vi "Begin.vi"() -> (0 "error out":errorcluster)   [LabVIEW 2013]
doc: "Called before other user functions, this VI is expected to open initial I/O refnums, load in file data, and do all program initialization. Notice that the <B>error out</B> terminal is simply used for data flow. Wiring it to other structures or subVIs ensures that this VI runs first."
uses:
  <vilib>/Rock Robotics/WPI/Joystick/WPI_JoystickDeviceEnum.ctl
  <vilib>/Rock Robotics/SystemInterfaces/Typedef/FPGA_TypedefDigitalModule.ctl
  <vilib>/Rock Robotics/SystemInterfaces/DIO/FPGA_DIOChannel.ctl
  <vilib>/Rock Robotics/SystemInterfaces/DIO/FPGA_DIORelayChannel.ctl
  <vilib>/Rock Robotics/SystemInterfaces/Typedef/FPGA_TypedefSolenoidModule.ctl
  <vilib>/Rock Robotics/WPI/Solenoid/WPI_SolenoidChannel.ctl
  <vilib>/Rock Robotics/WPI/Solenoid/WPI_SolenoidValue.ctl
  <vilib>/Rock Robotics/SystemInterfaces/DIO/FPGA_DIOPWMChannel.ctl
  <vilib>/Rock Robotics/WPI/Encoder/WPI_EncoderType.ctl
  <vilib>/Rock Robotics/WPI/Solenoid/WPI_SolenoidOpenDouble.vi
  <vilib>/Rock Robotics/WPI/Solenoid/WPI_SolenoidSetEnum.vi
  <vilib>/Rock Robotics/WPI/Counter/WPI_CounterDigitalInputToDigitalSource.vi
  <vilib>/Rock Robotics/WPI/RobotDrive/WPI_RobotDriveOpen2MotorWithVictor.vi
  <vilib>/Rock Robotics/WPI/MotorControl/WPI_MotorControlOpen Jaguar.vi
  <vilib>/Rock Robotics/WPI/MotorControl/WPI_MotorControlOpen Victor.vi
  <vilib>/Rock Robotics/WPI/Compressor/WPI_CompressorGetSetRefNum.vi
  <vilib>/Rock Robotics/WPI/Camera/WPI_CameraImageSize.ctl
  <vilib>/Rock Robotics/WPI/Camera/WPI_CameraWhite Balance Values.ctl
  <vilib>/Rock Robotics/WPI/Camera/WPI_CameraExposure Values.ctl
  <vilib>/Rock Robotics/WPI/Camera/WPI_CameraFrameRate.ctl
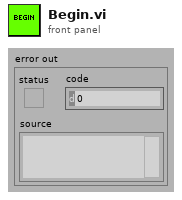
[diagram p1: front panel]
types:
  T1 = typedef "FPGA_DIOChannel.ctl" = enum8{"DIO 1", "DIO 2", "DIO 3", "DIO 4", "DIO 5", "DIO 6", "DIO 7", "DIO 8", "DIO 9", "DIO 10", "DIO 11", "DIO 12", "DIO 13", "DIO 14", "Invalid"}
  T2 = typedef "WPI_SolenoidChannel.ctl" = enum8{"Solenoid 1", "Solenoid 2", "Solenoid 3", "Solenoid 4", "Solenoid 5", "Solenoid 6", "Solenoid 7", "Solenoid 8", "Invalid"}
  T3 = typedef "FPGA_DIOPWMChannel.ctl" = enum8{"PWM 1", "PWM 2", "PWM 3", "PWM 4", "PWM 5", "PWM 6", "PWM 7", "PWM 8", "PWM 9", "PWM 10", "Invalid"}
  T4 = typedef "WPI_EncoderType.ctl" = enum16{"1x", "2x", "4x"}
  T5 = typedef "WPI_SolenoidValue.ctl" = enum16{"Off", "On", "Forward", "Reverse"}
  T6 = typedef "FPGA_TypedefSolenoidModule.ctl" = enum16{"Solenoid Module 1", "Solenoid Module 2"}
  T7 = typedef "FPGA_DIORelayChannel.ctl" = enum8{"Relay 1", "Relay 2", "Relay 3", "Relay 4", "Relay 5", "Relay 6", "Relay 7", "Relay 8", "Invalid"}
  T8 = typedef "WPI_JoystickDeviceEnum.ctl" = enum16{"USB 1", "USB 2", "USB 3", "USB 4", "Kinect 1", "Kinect 2"}
  T9 = typedef "FPGA_TypedefDigitalModule.ctl" = enum16{"Digital Module 1", "Digital Module 2"}
  T10 = typedef "WPI_CameraFrameRate.ctl" = u32
  T11 = typedef "WPI_CameraExposure Values.ctl" = enum16{"Auto", "Flicker-free 50 Hz", "Flicker-free 60 Hz", "Hold current"}
  T12 = typedef "WPI_CameraWhite Balance Values.ctl" = enum16{"Auto", "Fixed indoor", "Fixed outdoor 1", "Fixed outdoor 2", "Fixed fluorescent 1", "Fixed fluorescent 2", "Hold current"}
  T13 = typedef "WPI_CameraImageSize.ctl" = enum16{"640x480", "320x240", "160x120"}
  T14 = typedef "WPI_CameraDevRef.ctl" = cluster{"Camera Address":string, "CameraStatus":errorcluster, "Acquire Image Notifier":refnum<notifier>}
  T15 = typedef "WPI_DigitalInputDevRef.ctl" = cluster{"DevStatus":errorcluster, "DIO Channel":T1, "Digital Module":T9}
  T16 = typedef "WPI_MotorControlDeviceRef.ctl" = cluster{"DeviceStatus":errorcluster, "Type":enum16{"PWM", "CAN"}, "PWM":cluster{"Digital Module":T9, "PWM Channel":T3, "DeadBand":T17}, "CAN":cluster{"Device Number":u8, "Control Mode":T18, "Semaphore":T19, "Max Vout":dbl}, "Invert":bool, "TransformRef":T20, "InvTransformRef":T20}
  T17 = typedef "WPI_PWMDeadband.ctl" = cluster{"Name":string, "maxPositivePwm":i32, "minPositivePwm":i32, "centerPwm":i32, "maxNegativePwm":i32, "minNegativePwm":i32, "angularRange":u16}
  T18 = typedef "WPI_CANJaguar_ControlMode.ctl" = enum8{"Percent VBus", "Current", "Speed", "Position", "Voltage"}
  T19 = typedef "Semaphore RefNum" = refnum<k1>
  T20 = typedef "WPI_PWMTransform_ConPane.ctl" = refnum<vi>
  T21 = typedef "WPI_SolenoidDevRef.ctl" = cluster{"DevStatus":errorcluster, "Solenoid Module":T6, "Forward Solenoid Channel":T2, "Reverse Solenoid Channel":T2}
  T22 = typedef "FPGA_CounterEncoderSourceConvertionLVSourceType.ctl" = cluster{"DevStatus":errorcluster, "AnalogTriggerMode?":bool, "DigitalMode":cluster{"Digital Module":T9, "DIO Channel":T23}, "AnalogTriggerMode":cluster{"AnalogTriggerIndex":T24, "OutputType":T25}}
  T23 = typedef "FPGA_DIODigitalSourceChannel.ctl" = enum8{"DIO 1", "DIO 2", "DIO 3", "DIO 4", "DIO 5", "DIO 6", "DIO 7", "DIO 8", "DIO 9", "DIO 10", "DIO 11", "DIO 12", "DIO 13", "DIO 14", "Disabled"}
  T24 = typedef "FPGA_AnalogTriggerIndex.ctl" = enum8{"Trig 0", "Trig 1", "Trig 2", "Trig 3", "Trig 4", "Trig 5", "Trig 6", "Trig 7", "Invalid"}
  T25 = typedef "FPGA_AnalogTriggerOutType.ctl" = enum16{"InWindow", "TriggerState", "Rising", "Falling"}
  T26 = typedef "WPI_CompressorDevRef.ctl" = cluster{"DevStatus":errorcluster, "DigitalInputDevRef":T15, "RelayDevRef":T27}
  T27 = typedef "WPI_RelayDevRef.ctl" = cluster{"DevStatus":errorcluster, "Relay Channel":T7, "Digital Module":T9, "Relay Direction":T28}
  T28 = typedef "WPI_RelayDirection.ctl" = enum16{"Both directions", "Forward only", "Reverse only"}
  T29 = typedef "WPI_RobotDriveDevRef.ctl" = cluster{"DevStatus":errorcluster, "Motors[]":T16[], "Square Inputs":bool, "Max Output":dbl, "Isochronous":bool}
  T30 = typedef "WPI_EncoderDevRef.ctl" = cluster{"DevStatus":errorcluster, "EncoderIndex":T31, "CounterIndex":T32, "DistancePerCount":dbl, "Decoding Type":T4}
  T31 = typedef "FPGA_EncoderIdx.ctl" = enum8{"Enc 0", "Enc 1", "Enc 2", "Enc 3", "Invalid"}
  T32 = typedef "FPGA_CounterCtrSystemIndex.ctl" = enum8{"Ctr 0", "Ctr 1", "Ctr 2", "Ctr 3", "Ctr 4", "Ctr 5", "Ctr 6", "Ctr 7", "Invalid"}
  T33 = typedef "WPI_JoystickDevRef.ctl" = cluster{"Device":T8}
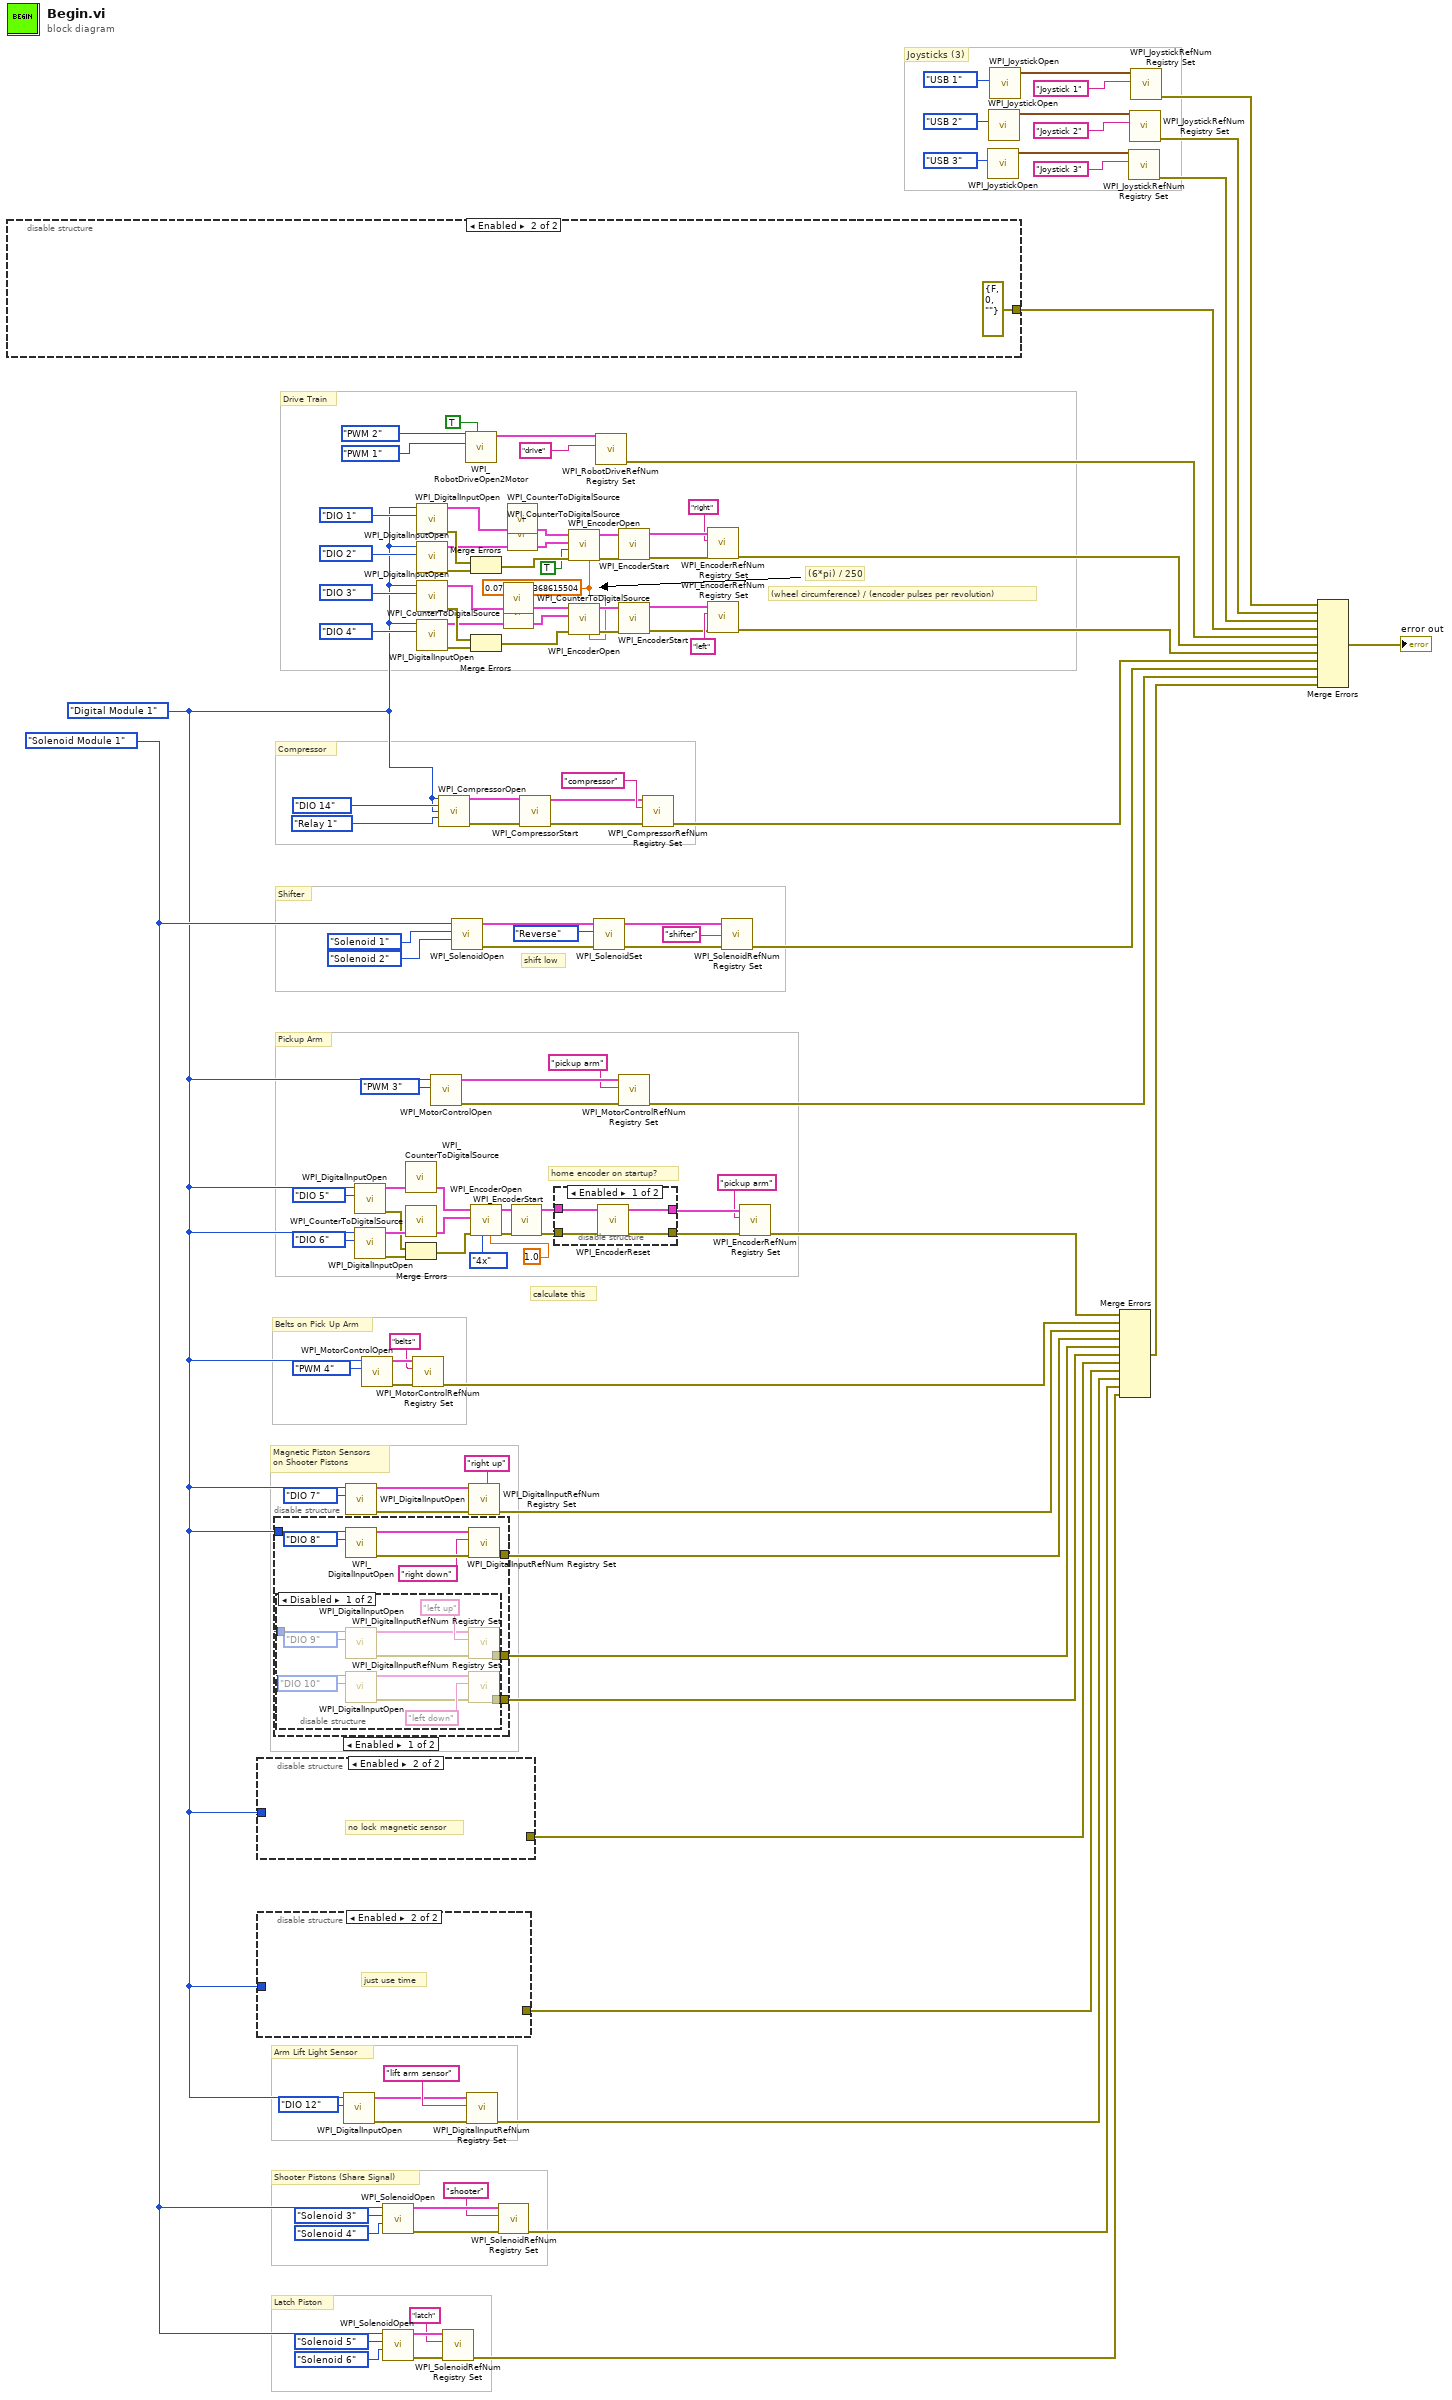
[diagram p0: block diagram]
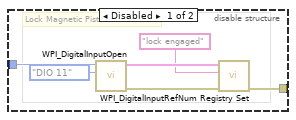
[diagram p2: hidden frame]
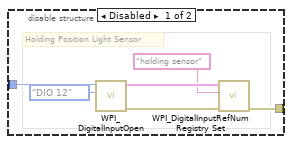
[diagram p5: hidden frame]
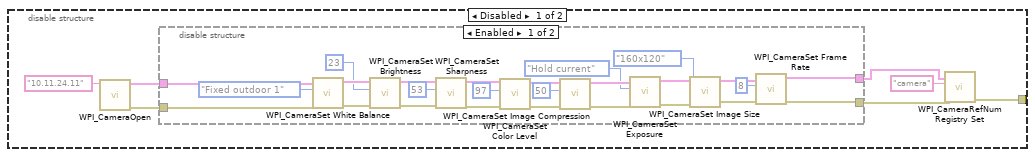
[diagram p7: hidden frame]
diagram:
  w72 = 0.07539822368615504 ("DistancePerCount")
  w13 = FPGA_TypedefSolenoidModule."Solenoid Module 1" ("Solenoid Module (Module 1)")
  w6 = FPGA_TypedefDigitalModule."Digital Module 1" ("Digital Module (Module 1)")
  # "Arm Lift Light Sensor"
  # "Joysticks (3)"
  # "Latch Piston"
  # "Shooter Pistons (Share Signal)"
  # "Magnetic Piston Sensors\non Shooter Pistons"
  # "Belts on Pick Up Arm"
  # "calculate this"
  # "Pickup Arm"
  # "home encoder on startup?"
  # "Shifter"
  # "Compressor"
  # "Drive Train"
  # "shift low"
  # "(wheel circumference) / (encoder pulses per revolution)"
  # "(6*pi) / 250"
  n1 = disable-structure shown="Enabled" {
    disable-tunnel: [w129 errorcluster {"status"=FALSE, "code"=0, "source"=""} ("error out")] -> w116
    frame Disabled {
      n2 = call <vilib>:"WPI_CameraOpen.vi"("Camera Address"="10.11.24.11") -> ("error out"=w131:errorcluster, "CameraDevRef"=w133:T14)  [unwired: 9 in]
      n3 = disable-structure shown="Enabled" {
        disable-tunnel: w133 -> [w159 w163]
        disable-tunnel: [w137 w163] -> w132
        disable-tunnel: w131 -> [w146 w162]
        disable-tunnel: [w136 w162] -> w130
        frame Enabled {
          n4 = call <vilib>:"WPI_CameraSet White Balance.vi"("error in (no error)"=w146, "White Balance"=WPI_CameraWhite_Balance_Values."Fixed outdoor 1", "CameraDevRef"=w159) -> ("error out"=w147:errorcluster, "CameraDevRef Out"=w158:T14)  [unwired: 7 in]
          n5 = call <vilib>:"WPI_CameraSet Brightness.vi"("error in (no error)"=w147, "Brightness"=23, "CameraDevRef"=w158) -> ("error out"=w148:errorcluster, "CameraDevRef Out"=w157:T14)  [unwired: 7 in]
          n6 = call <vilib>:"WPI_CameraSet Sharpness.vi"("error in (no error)"=w148, "Sharpness"=53, "CameraDevRef"=w157) -> ("error out"=w149:errorcluster, "CameraDevRef Out"=w156:T14)  [unwired: 7 in]
          n7 = call <vilib>:"WPI_CameraSet Color Level.vi"("error in (no error)"=w149, "Color Level"=97, "CameraDevRef"=w156) -> ("error out"=w150:errorcluster, "CameraDevRef Out"=w155:T14)  [unwired: 7 in]
          n8 = call <vilib>:"WPI_CameraSet Image Compression.vi"("error in (no error)"=w150, "Compression"=50, "CameraDevRef"=w155) -> ("error out"=w161:errorcluster, "CameraDevRef Out"=w160:T14)  [unwired: 7 in]
          n9 = call <vilib>:"WPI_CameraSet Exposure.vi"("error in (no error)"=w161, "Exposure"=WPI_CameraExposure_Values."Hold current", "CameraDevRef"=w160) -> ("error out"=w151:errorcluster, "CameraDevRef Out"=w154:T14)  [unwired: 7 in]
          n10 = call <vilib>:"WPI_CameraSet Image Size.vi"("error in (no error)"=w151, "Image Size"=WPI_CameraImageSize."160x120", "CameraDevRef"=w154) -> ("error out"=w152:errorcluster, "CameraDevRef Out"=w153:T14)  [unwired: 7 in]
          n11 = call <vilib>:"WPI_CameraSet Frame Rate.vi"("error in (no error)"=w152, "Frame Rate (fps)"=T10 8, "CameraDevRef"=w153) -> ("error out"=w136:errorcluster, "CameraDevRef Out"=w137:T14)  [unwired: 7 in]
        }
        frame Disabled {
        }
      }
      n12 = call <vilib>:"WPI_CameraRefNum Registry Set.vi"("error in (no error)"=w130, "refnum name"="camera", "CameraDevRef"=w132) -> ("error out"=w129:errorcluster)  [unwired: 7 in, 1 out]
    }
    frame Enabled {
    }
  }
  n13 = disable-structure shown="Enabled" {
    disable-tunnel: w6 -> [w166 _]
    disable-tunnel: [w165 _] -> w1
    frame Disabled {
      # "Lock Magnetic Piston Sensor"
      n14 = call <vilib>:"WPI_DigitalInputOpen.vi"("DIO Channel"=FPGA_DIOChannel."DIO 11", "Digital Module (Module 1)"=w166) -> ("error out"=w169:errorcluster, "DigitalInputDevRef"=w168:T15)  [unwired: 8 in]
      n15 = call <vilib>:"WPI_DigitalInputRefNum Registry Set.vi"("error in (no error)"=w169, "refnum name"="lock engaged", "DigitalInputDevRef"=w168) -> ("error out"=w165:errorcluster)  [unwired: 7 in, 1 out]
    }
    frame Enabled {
      # "no lock magnetic sensor"
    }
  }
  n16 = disable-structure shown="Enabled" {
    disable-tunnel: w6 -> [w172 _]
    disable-tunnel: [w171 _] -> w2
    frame Disabled {
      # "Holding Position Light Sensor"
      n17 = call <vilib>:"WPI_DigitalInputOpen.vi"("DIO Channel"=FPGA_DIOChannel."DIO 12", "Digital Module (Module 1)"=w172) -> ("error out"=w175:errorcluster, "DigitalInputDevRef"=w174:T15)  [unwired: 8 in]
      n18 = call <vilib>:"WPI_DigitalInputRefNum Registry Set.vi"("error in (no error)"=w175, "refnum name"="holding sensor", "DigitalInputDevRef"=w174) -> ("error out"=w171:errorcluster)  [unwired: 7 in, 1 out]
    }
    frame Enabled {
      # "just use time"
    }
  }
  n19 = disable-structure shown="Enabled" {
    disable-tunnel: [w181 _] -> w24
    disable-tunnel: w6 -> [w179 _]
    disable-tunnel: [w178 _] -> w8
    disable-tunnel: [w177 _] -> w7
    frame Enabled {
      n20 = disable-structure shown="Disabled" {
        disable-tunnel: w179 -> [w187 _]
        disable-tunnel: [w186 _] -> w178
        disable-tunnel: [w185 _] -> w177
        frame Disabled {
          n21 = call <vilib>:"WPI_DigitalInputOpen.vi"("DIO Channel"=FPGA_DIOChannel."DIO 9", "Digital Module (Module 1)"=w187) -> ("error out"=w188:errorcluster, "DigitalInputDevRef"=w189:T15)  [unwired: 8 in]
          n22 = call <vilib>:"WPI_DigitalInputOpen.vi"("DIO Channel"=FPGA_DIOChannel."DIO 10", "Digital Module (Module 1)"=w187) -> ("error out"=w190:errorcluster, "DigitalInputDevRef"=w191:T15)  [unwired: 8 in]
          n23 = call <vilib>:"WPI_DigitalInputRefNum Registry Set.vi"("error in (no error)"=w188, "refnum name"="left up", "DigitalInputDevRef"=w189) -> ("error out"=w186:errorcluster)  [unwired: 7 in, 1 out]
          n24 = call <vilib>:"WPI_DigitalInputRefNum Registry Set.vi"("error in (no error)"=w190, "refnum name"="left down", "DigitalInputDevRef"=w191) -> ("error out"=w185:errorcluster)  [unwired: 7 in, 1 out]
        }
        frame Enabled {
        }
      }
      n25 = call <vilib>:"WPI_DigitalInputOpen.vi"("DIO Channel"=FPGA_DIOChannel."DIO 8", "Digital Module (Module 1)"=w179) -> ("error out"=w184:errorcluster, "DigitalInputDevRef"=w183:T15)  [unwired: 8 in]
      n26 = call <vilib>:"WPI_DigitalInputRefNum Registry Set.vi"("error in (no error)"=w184, "refnum name"="right down", "DigitalInputDevRef"=w183) -> ("error out"=w181:errorcluster)  [unwired: 7 in, 1 out]
    }
    frame Disabled {
      # "dang, only one sensor\non the pistons..."
    }
  }
  n27 = call <vilib>:"WPI_DigitalInputOpen.vi"("DIO Channel"=FPGA_DIOChannel."DIO 12", "Digital Module (Module 1)"=w6) -> ("error out"=w10:errorcluster, "DigitalInputDevRef"=w11:T15)  [unwired: 8 in]
  n28 = call <vilib>:"WPI_DigitalInputOpen.vi"("DIO Channel"=FPGA_DIOChannel."DIO 7", "Digital Module (Module 1)"=w6) -> ("error out"=w29:errorcluster, "DigitalInputDevRef"=w28:T15)  [unwired: 8 in]
  n29 = call <vilib>:"WPI_DigitalInputOpen.vi"("DIO Channel"=FPGA_DIOChannel."DIO 5", "Digital Module (Module 1)"=w6) -> ("error out"=w47:errorcluster, "DigitalInputDevRef"=w52:T15)  [unwired: 8 in]
  n30 = call <vilib>:"WPI_DigitalInputOpen.vi"("DIO Channel"=FPGA_DIOChannel."DIO 6", "Digital Module (Module 1)"=w6) -> ("error out"=w48:errorcluster, "DigitalInputDevRef"=w51:T15)  [unwired: 8 in]
  n31 = call-poly <vilib>:"WPI_MotorControlOpen.vi"("PWM Channel"=FPGA_DIOPWMChannel."PWM 4", "Digital Module (Module 1)"=w6) -> ("error out"=w35:errorcluster, "MotorControlDeviceRef"=w34:T16)  [unwired: 8 in]
  n32 = call-poly <vilib>:"WPI_SolenoidOpen.vi"("Reverse Solenoid Channel"=WPI_SolenoidChannel."Solenoid 4", "Forward Solenoid Channel"=WPI_SolenoidChannel."Solenoid 3", "Solenoid Module (Module 1)"=w13) -> ("error out"=w19:errorcluster, "SolenoidDevRef"=w18:T21)  [unwired: 7 in]
  n33 = call-poly <vilib>:"WPI_SolenoidOpen.vi"("Reverse Solenoid Channel"=WPI_SolenoidChannel."Solenoid 6", "Forward Solenoid Channel"=WPI_SolenoidChannel."Solenoid 5", "Solenoid Module (Module 1)"=w13) -> ("error out"=w17:errorcluster, "SolenoidDevRef"=w16:T21)  [unwired: 7 in]
  n34 = call-poly <vilib>:"WPI_CounterToDigitalSource.vi"("DigitalInputDevRef"=w52) -> ("Digital Source"=w50:T22)  [unwired: 6 in]
  n35 = call-poly <vilib>:"WPI_CounterToDigitalSource.vi"("DigitalInputDevRef"=w51) -> ("Digital Source"=w49:T22)  [unwired: 6 in]
  n36 = Merge Errors(w47, w48) -> (w46:errorcluster)
  n37 = call <vilib>:"WPI_MotorControlRefNum Registry Set.vi"("error in (no error)"=w35, "refnum name"="belts", "MotorControlDevRef"=w34) -> ("error out"=w32:errorcluster)  [unwired: 7 in, 1 out]
  n38 = call <vilib>:"WPI_DigitalInputOpen.vi"("DIO Channel"=FPGA_DIOChannel."DIO 1", "Digital Module (Module 1)"=w6) -> ("error out"=w66:errorcluster, "DigitalInputDevRef"=w80:T15)  [unwired: 8 in]
  n39 = call <vilib>:"WPI_DigitalInputOpen.vi"("DIO Channel"=FPGA_DIOChannel."DIO 2", "Digital Module (Module 1)"=w6) -> ("error out"=w68:errorcluster, "DigitalInputDevRef"=w65:T15)  [unwired: 8 in]
  n40 = call <vilib>:"WPI_DigitalInputOpen.vi"("DIO Channel"=FPGA_DIOChannel."DIO 3", "Digital Module (Module 1)"=w6) -> ("error out"=w69:errorcluster, "DigitalInputDevRef"=w94:T15)  [unwired: 8 in]
  n41 = call <vilib>:"WPI_DigitalInputOpen.vi"("DIO Channel"=FPGA_DIOChannel."DIO 4", "Digital Module (Module 1)"=w6) -> ("error out"=w71:errorcluster, "DigitalInputDevRef"=w64:T15)  [unwired: 8 in]
  n42 = call-poly <vilib>:"WPI_MotorControlOpen.vi"("PWM Channel"=FPGA_DIOPWMChannel."PWM 3", "Digital Module (Module 1)"=w6) -> ("error out"=w59:errorcluster, "MotorControlDeviceRef"=w58:T16)  [unwired: 8 in]
  n43 = call <vilib>:"WPI_CompressorOpen.vi"("Pressure Switch Digital Module (Module 1)"=w6, "Pressure Switch DIO Channel"=FPGA_DIOChannel."DIO 14", "Relay Digital Module (Module 1)"=w6, "Relay Channel"=FPGA_DIORelayChannel."Relay 1") -> ("CompressorDevRef"=w108:T26, "error out"=w107:errorcluster)  [unwired: 10 in]
  n44 = call <vilib>:"WPI_SolenoidRefNum Registry Set.vi"("error in (no error)"=w17, "refnum name"="latch", "SolenoidDevRef"=w16) -> ("error out"=w5:errorcluster)  [unwired: 7 in, 1 out]
  n45 = call-poly <vilib>:"WPI_SolenoidOpen.vi"("Reverse Solenoid Channel"=WPI_SolenoidChannel."Solenoid 2", "Forward Solenoid Channel"=WPI_SolenoidChannel."Solenoid 1", "Solenoid Module (Module 1)"=w13) -> ("error out"=w99:errorcluster, "SolenoidDevRef"=w100:T21)  [unwired: 7 in]
  n46 = call-poly <vilib>:"WPI_RobotDriveOpen2Motor.vi"("Left Motor Inverted"=TRUE, "Right Motor"=FPGA_DIOPWMChannel."PWM 1", "Left Motor"=FPGA_DIOPWMChannel."PWM 2") -> ("RobotDriveDevRef"=w96:T29)  [unwired: 7 in, 1 out]
  n47 = call <vilib>:"WPI_DigitalInputRefNum Registry Set.vi"("error in (no error)"=w10, "refnum name"="lift arm sensor", "DigitalInputDevRef"=w11) -> ("error out"=w3:errorcluster)  [unwired: 7 in, 1 out]
  n48 = call <vilib>:"WPI_DigitalInputRefNum Registry Set.vi"("error in (no error)"=w29, "refnum name"="right up", "DigitalInputDevRef"=w28) -> ("error out"=w25:errorcluster)  [unwired: 7 in, 1 out]
  n49 = Merge Errors(w66, w68) -> (w67:errorcluster)
  n50 = Merge Errors(w69, w71) -> (w70:errorcluster)
  n51 = call <vilib>:"WPI_EncoderOpen.vi"("DistancePerCount"=1.0, "Decoding Type"=WPI_EncoderType."4x", "error in (no error)"=w46, "BSource"=w49, "ASource"=w50) -> ("error out"=w45:errorcluster, "EncoderDevRef"=w44:T30)  [unwired: 5 in]
  n52 = call <vilib>:"WPI_SolenoidRefNum Registry Set.vi"("error in (no error)"=w19, "refnum name"="shooter", "SolenoidDevRef"=w18) -> ("error out"=w4:errorcluster)  [unwired: 7 in, 1 out]
  n53 = call-poly <vilib>:"WPI_CounterToDigitalSource.vi"("DigitalInputDevRef"=w94) -> ("Digital Source"=w87:T22)  [unwired: 6 in]
  n54 = call-poly <vilib>:"WPI_CounterToDigitalSource.vi"("DigitalInputDevRef"=w64) -> ("Digital Source"=w88:T22)  [unwired: 6 in]
  n55 = call-poly <vilib>:"WPI_CounterToDigitalSource.vi"("DigitalInputDevRef"=w80) -> ("Digital Source"=w86:T22)  [unwired: 6 in]
  n56 = call-poly <vilib>:"WPI_CounterToDigitalSource.vi"("DigitalInputDevRef"=w65) -> ("Digital Source"=w85:T22)  [unwired: 6 in]
  n57 = call <vilib>:"WPI_EncoderStart.vi"("error in (no error)"=w45, "EncoderDevRef"=w44) -> ("error out"=w43:errorcluster, "EncoderDevRef"=w42:T30)  [unwired: 8 in]
  n58 = call <vilib>:"WPI_CompressorStart.vi"("error in (no error)"=w107, "CompressorDevRef"=w108) -> ("error out"=w106:errorcluster, "CompressorDevRef"=w105:T26)  [unwired: 8 in]
  n59 = disable-structure shown="Enabled" {
    disable-tunnel: w43 -> [w199 w200]
    disable-tunnel: w42 -> [w198 w201]
    disable-tunnel: [w197 w201] -> w40
    disable-tunnel: [w196 w200] -> w41
    frame Enabled {
      n60 = call <vilib>:"WPI_EncoderReset.vi"("error in (no error)"=w199, "EncoderDevRef"=w198) -> ("error out"=w196:errorcluster, "EncoderDevRef"=w197:T30)  [unwired: 8 in]
    }
    frame Disabled {
    }
  }
  n61 = call <vilib>:"WPI_EncoderOpen.vi"("DistancePerCount"=w72, "error in (no error)"=w67, "Invert Direction (False)"=TRUE, "BSource"=w85, "ASource"=w86) -> ("error out"=w84:errorcluster, "EncoderDevRef"=w83:T30)  [unwired: 5 in]
  n62 = call <vilib>:"WPI_EncoderOpen.vi"("DistancePerCount"=w72, "error in (no error)"=w70, "BSource"=w88, "ASource"=w87) -> ("error out"=w89:errorcluster, "EncoderDevRef"=w90:T30)  [unwired: 6 in]
  n63 = call-poly <vilib>:"WPI_SolenoidSet.vi"("error in (no error)"=w99, "Value"=WPI_SolenoidValue."Reverse", "SolenoidDevRef"=w100) -> ("error out"=w98:errorcluster, "SolenoidDevRef"=w97:T21)  [unwired: 7 in]
  n64 = call <vilib>:"WPI_RobotDriveRefNum Registry Set.vi"("refnum name"="drive", "RobotDriveDevRef"=w96) -> ("error out"=w115:errorcluster)  [unwired: 8 in, 1 out]
  n65 = call <vilib>:"WPI_EncoderStart.vi"("error in (no error)"=w84, "EncoderDevRef"=w83) -> ("error out"=w82:errorcluster, "EncoderDevRef"=w81:T30)  [unwired: 8 in]
  n66 = call <vilib>:"WPI_EncoderStart.vi"("error in (no error)"=w89, "EncoderDevRef"=w90) -> ("error out"=w91:errorcluster, "EncoderDevRef"=w92:T30)  [unwired: 8 in]
  n67 = call <vilib>:"WPI_MotorControlRefNum Registry Set.vi"("error in (no error)"=w59, "refnum name"="pickup arm", "MotorControlDevRef"=w58) -> ("error out"=w55:errorcluster)  [unwired: 7 in, 1 out]
  n68 = call <vilib>:"WPI_CompressorRefNum Registry Set.vi"("error in (no error)"=w106, "refnum name"="compressor", "CompressorDevRef"=w105) -> ("error out"=w60:errorcluster)  [unwired: 7 in, 1 out]
  n69 = call <vilib>:"WPI_EncoderRefNum Registry Set.vi"("error in (no error)"=w82, "refnum name"="right", "EncoderDevRef"=w81) -> ("error out"=w114:errorcluster)  [unwired: 7 in, 1 out]
  n70 = call <vilib>:"WPI_EncoderRefNum Registry Set.vi"("error in (no error)"=w91, "refnum name"="left", "EncoderDevRef"=w92) -> ("error out"=w113:errorcluster)  [unwired: 7 in, 1 out]
  n71 = call <vilib>:"WPI_SolenoidRefNum Registry Set.vi"("error in (no error)"=w98, "refnum name"="shifter", "SolenoidDevRef"=w97) -> ("error out"=w61:errorcluster)  [unwired: 7 in, 1 out]
  n72 = call <vilib>:"WPI_EncoderRefNum Registry Set.vi"("error in (no error)"=w41, "refnum name"="pickup arm", "EncoderDevRef"=w40) -> ("error out"=w31:errorcluster)  [unwired: 7 in, 1 out]
  n73 = call <vilib>:"WPI_JoystickOpen.vi"("JoystickDevice"=WPI_JoystickDeviceEnum."USB 3") -> ("JoystickDevRef"=w127:T33)  [unwired: 10 in]
  n74 = call <vilib>:"WPI_JoystickOpen.vi"("JoystickDevice"=WPI_JoystickDeviceEnum."USB 2") -> ("JoystickDevRef"=w124:T33)  [unwired: 10 in]
  n75 = call <vilib>:"WPI_JoystickOpen.vi"("JoystickDevice"=WPI_JoystickDeviceEnum."USB 1") -> ("JoystickDevRef"=w121:T33)  [unwired: 10 in]
  n76 = Merge Errors(w31, w32, w25, w24, w8, w7, w1, w2, w3, w4, w5) -> (w30:errorcluster)
  n77 = call <vilib>:"WPI_JoystickRefNum Registry Set.vi"("refnum name"="Joystick 3", "JoystickDevRef"=w127) -> ("error out"=w117:errorcluster)  [unwired: 8 in, 1 out]
  n78 = call <vilib>:"WPI_JoystickRefNum Registry Set.vi"("refnum name"="Joystick 2", "JoystickDevRef"=w124) -> ("error out"=w118:errorcluster)  [unwired: 8 in, 1 out]
  n79 = call <vilib>:"WPI_JoystickRefNum Registry Set.vi"("refnum name"="Joystick 1", "JoystickDevRef"=w121) -> ("error out"=w119:errorcluster)  [unwired: 8 in, 1 out]
  n80 = Merge Errors(w119, w118, w117, w116, w115, w114, w113, w60, w61, w55, w30) -> (→"error out":errorcluster)
